vi "CalcPossibleTurretMoves.vi"(10 "Setpoint Direction":dbl, 11 "Turret Angle":dbl) -> (3 "Possible Turet Angle Changes":dbl[](array[numeric]))   [LabVIEW 2014]
uses:
  <vilib>/Analysis/coordinate.llb/Angle Range (Degree).ctl
  <vilib>/Analysis/coordinate.llb/Wrap Angle (scalar).vi
  <vilib>/Analysis/NI_AAL_Angle.lvlib
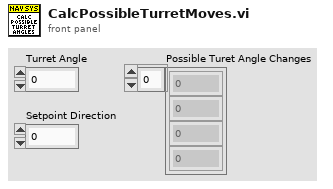
[diagram p1: front panel]
types:
  T1 = typedef "NI_AAL_Angle.lvlib/Angle Range (Degree).ctl" = u16
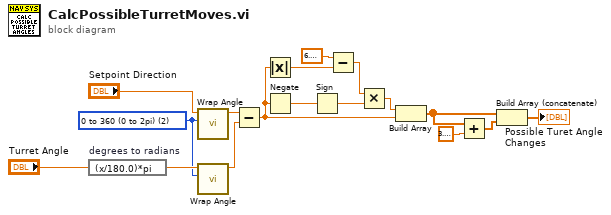
[diagram p0: block diagram]
diagram:
  w14 = T1 2 items=["none", "-180 to 180 (-pi to pi)", "0 to 360 (0 to 2pi)"] ("angle range")
  n1 = expression code="(x/180.0)*pi" "degrees to radians"("Turret Angle") -> (w15:dbl)
  n2 = call-poly <vilib>:"Wrap Angle.vi"("angle range"=w14, "angle in"="Setpoint Direction") -> ("angle out"=w13:dbl)  [unwired: 8 in, 1 out]
  n3 = call-poly <vilib>:"Wrap Angle.vi"("angle range"=w14, "angle in"=w15) -> ("angle out"=w12:dbl)  [unwired: 8 in, 1 out]
  n4 = Subtract(x=w13, y=w12) -> (x-y=w5:dbl)
  n5 = Absolute Value(x=w5) -> (abs(x)=w10:dbl)
  n6 = Negate(x=w5) -> (-x=w7:dbl)
  n7 = Sign(1:w7) -> (0:w8:dbl)
  n8 = Subtract(x=6.283185307179586, y=w10) -> (x-y=w9:dbl)
  n9 = Multiply(x=w9, y=w8) -> (x*y=w6:dbl)
  n10 = Build Array(w6, w5) -> (w2:dbl[])
  n11 = Add(x=w2, y=3.141592653589793) -> (x+y=w3:dbl[])
  n12 = Build Array (concatenate)(w2, w3) -> (→"Possible Turet Angle Changes":dbl[])
